vi "stringConvertToDate_yymmdd.vi"(1 "input_str_yymmdd":string) -> (0 "show_date":timestamp)   [LabVIEW 2011]
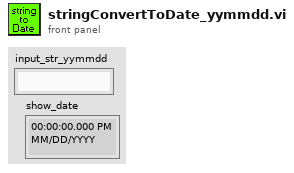
[diagram p1: front panel]
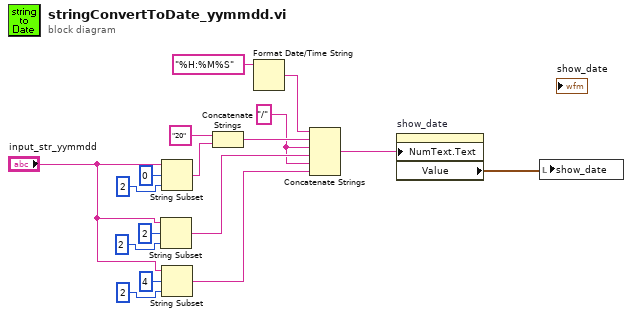
[diagram p0: block diagram]
diagram:
  w7 = "/"
  n1 = String Subset(string="input_str_yymmdd", offset (0)=2 ("偏移量(0)"), length (rest)=2 ("长度（剩余）")) -> (substring=w8:string)
  n2 = String Subset(string="input_str_yymmdd", offset (0)=0 ("偏移量(0)"), length (rest)=2 ("长度（剩余）")) -> (substring=w14:string)
  n3 = String Subset(string="input_str_yymmdd", offset (0)=4 ("偏移量(0)"), length (rest)=2 ("长度（剩余）")) -> (substring=w6:string)
  n4 = Concatenate Strings("20", w14) -> (w9:string)
  n5 = Format Date/Time String(time format string (%c)="%H:%M%S" ("时间格式字符串(%c)")) -> (date/time string=w4:string)  [unwired: 2 in]
  n6 = Concatenate Strings(w4, w9, w7, w8, w7, w6) -> (w3:string)
  n7 = property on="show_date" class="AbsTime (严格)"("NumText.Text"=w3) -> ("Value"=w2:timestamp)  [unwired: 2 in, 2 out]
  n8 = local write "show_date"(w2) -> ()
